vi "GetFixtureID.vi"(8 "error in (no error)":errorcluster, 10 "Current Fixture ID :":string="MEScannerFixture1") -> (0 "error out":errorcluster, 2 "Fixture Serial Number":string="MEScannerFixture1", 3 "OK":bool)   [LabVIEW 2015]
uses:
  <vilib>/Utility/miscctls.llb/LVSelectionTypeDef.ctl
panel:
  in  "Cancel Button":bool
  in  "OK Button":bool
  in  "Enter Fixture ID":string
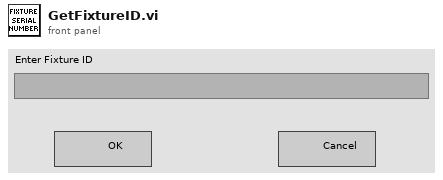
[diagram p1: front panel]
types:
  T1 = typedef "LVSelectionTypeDef.ctl" = cluster{"Selection Start":u32, "Selection End":u32}
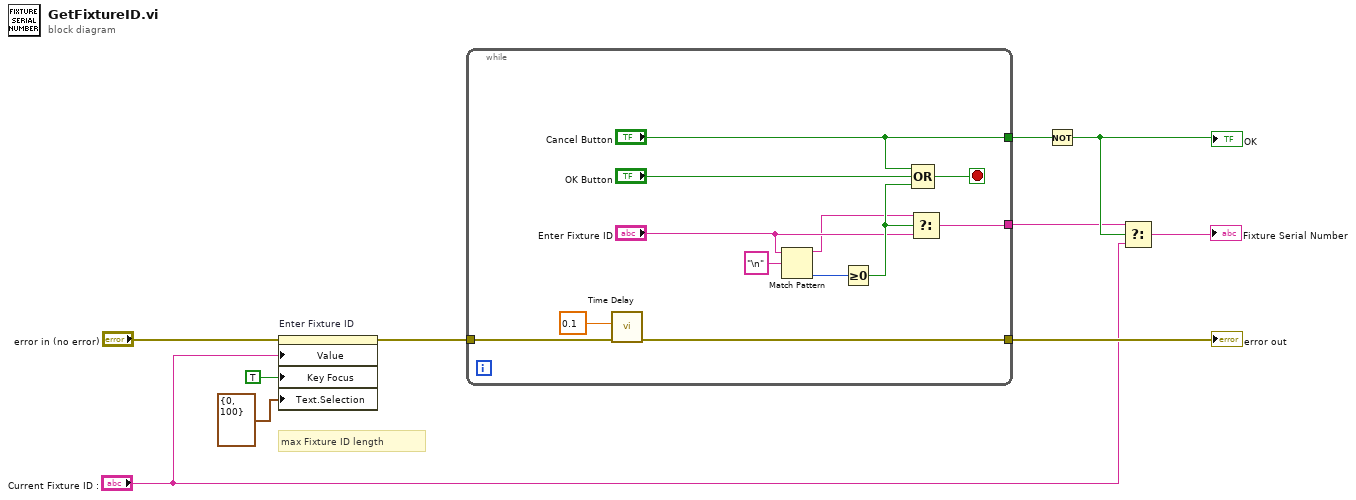
[diagram p0: block diagram]
diagram:
  # "max Fixture ID length"
  n1 = property on="Enter Fixture ID" class="Str"(error in="error in (no error)", "Value"="Current Fixture ID :", "Key Focus"=TRUE, "Text.Selection"=T1 {"Selection Start"=0, "Selection End"=100}) -> (error out=w4:errorcluster)  [unwired: 1 in, 1 out]
  n2 = while {
    tunnel: [w22] -> w10
    tunnel: w4 -> [w21]
    tunnel: [w13] -> w6
    tunnel: ["Cancel Button"] -> w9
    stop <- w18 stop-if-true
    n3 = call "Time Delay"("error in (no error)"=w21, "Delay Time (s)"=0.1) -> ("error out"=w22:errorcluster)  [unwired: 9 in]
    n4 = Match Pattern(string="Enter Fixture ID", regular expression="\n") -> (before substring=w11:string, offset past match=w19:i32)  [unwired: 1 in, 2 out]
    n5 = Greater Or Equal To 0?(x=w19) -> (x >= 0?=w15:bool)
    n6 = Select(t=w11, s=w15, f="Enter Fixture ID") -> (s? t:f=w13:string)
    n7 = Compound Arithmetic op=OR("Cancel Button", "OK Button", w15) -> (w18:bool)
  }
  "error out" <- w10
  n8 = Not(x=w9) -> (.not. x?=w8:bool)
  "OK" <- w8
  n9 = Select(t=w6, s=w8, f="Current Fixture ID :") -> (s? t:f=→"Fixture Serial Number":string)
